vi "PRUEBA_NEO.vi"() -> ()   [LabVIEW 2025]
panel:
  out "error out":errorcluster
  in  "Color Box":u32(colorbox)
  in  "stop":bool
  in  "VISA resource name":refnum<visa-resource-name>
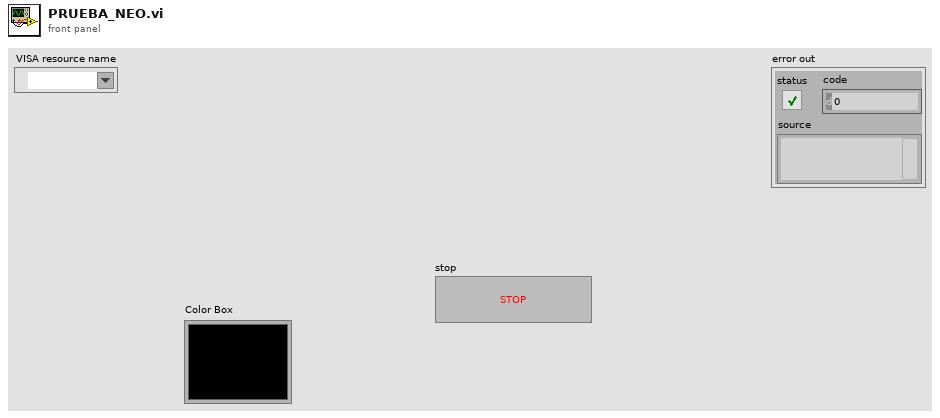
[diagram p1: front panel]
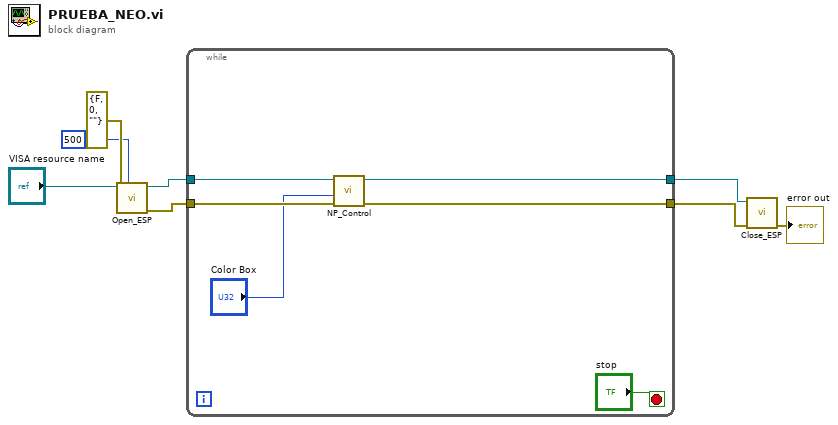
[diagram p0: block diagram]
diagram:
  n1 = call "Open_ESP.vi"("timeout (10sec)"=u32 500, "error in (no error)"=errorcluster {"status"=FALSE, "code"=0, "source"=""}, "VISA resource name"="VISA resource name") -> ("error out"=w3:errorcluster, "VISA resource name out"=w8:refnum<visa-resource-name>)  [unwired: 7 in]
  n2 = while {
    tunnel: w3 -> [w11]
    tunnel: [w13] -> w5
    tunnel: w8 -> [w14]
    tunnel: [w12] -> w4
    stop <- "stop" stop-if-true
    n3 = call "NP_Control.vi"("error in (no error)"=w11, "Color Box"="Color Box", "VISA resource name"=w14) -> ("error out"=w13:errorcluster, "VISA resource name out"=w12:refnum<visa-resource-name>)  [unwired: 7 in]
  }
  n4 = call "Close_ESP.vi"("error in (no error)"=w5, "VISA resource name"=w4) -> ("error out"=→"error out":errorcluster)  [unwired: 9 in]
